vi "2023_day13_Task2.vi"() -> ()   [LabVIEW 2021]
panel:
  out "Task 2":i32
  in  "Switch":bool caption="Ex. Data  vs.  User Data"
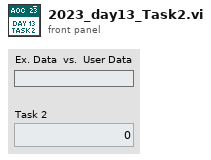
[diagram p1: front panel]
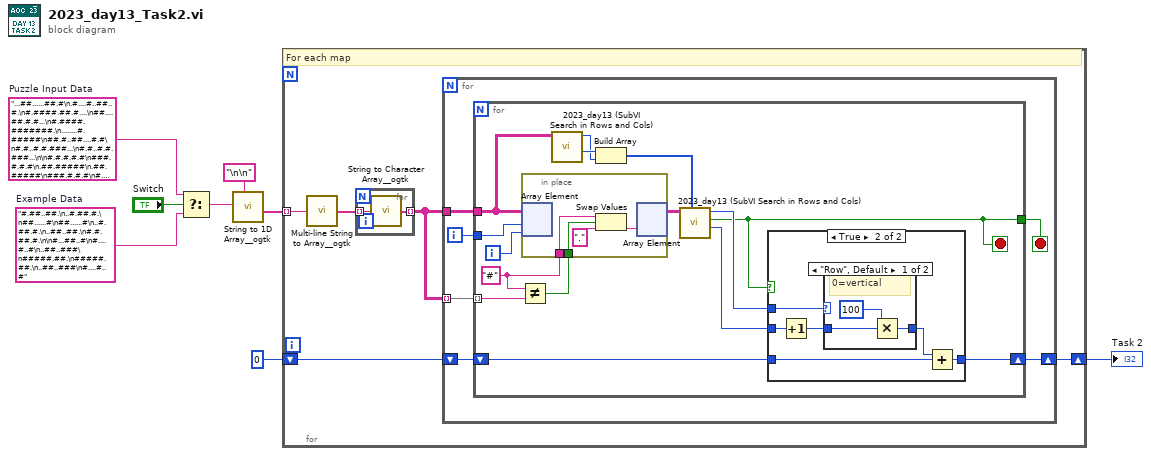
[diagram p0: block diagram]
diagram:
  w6 = "...##......##.#\n.#....#..##..#.\n#.####.##.#....\n##....##.#.#...\n#.####.#######.\n........#.#####\n##.#..##....#.#\n#.#..#.#.###...\n#.#..#.#.###...\n\n#.#.#.#.#\n###.#.#.#\n.##.#####\n.##.#####\n###.#.#.#\n#.#.#.#.#\n.#.##.#.#\n#.#..#..#\n..###.#..\n#..#.#.#.\n##.#...#.\n\n##.....#...\n##.....#...\n#..###....#\n##.#..#.##.\n#..#####..#\n#.#....#.#.\n.##.##....#\n.###..###.#\n...#.......\n....#.#.###\n#......#.##\n...#.##....\n...#.##....\n#......#.##\n....#.#.###\n...#.......\n.###..#####\n\n..####....#\n..####....#\n..#....#.##\n.....#.#..#\n#.#...##...\n###.###.##.\n..#..#...##\n..#..#...##\n###.###.##.\n#.#...##...\n.....#.#..#\n..#.#..#.##\n..####....#\n\n#.#####..\n#..#.#.#.\n.##.#..#.\n.##...##.\n.....#.##\n........#\n........#\n\n..#.###.##..#\n.##.###.##..#\n.#...#.#.#.##\n.#...#.#.#.##\n.##.###.##..#\n..#.###.##..#\n...#.#####.#.\n##.#...######\n..#..#..##.#.\n#..####.###.#\n.##..#....###\n\n####.##....\n....##.##.#\n...##...##.\n##..#..#..#\n##..#....#.\n##..#....#.\n##..#..#..#\n...##...##.\n....##.##.#\n####.##....\n##..#####..\n#..#....#..\n...#.....##\n....#####..\n########...\n#######.#.#\n####.#.#...\n\n..##.......\n#..##.#..#.\n.##....##..\n.#####....#\n#######..##\n.#...##..##\n..####.##.#\n#####..##..\n##.....##..\n##.....##..\n.####..##..\n\n#.#..###.#.##.#\n##.##.###.#..#.\n##...#..#......\n.##...##...##..\n##...###.#.##.#\n.##...#..######\n.#.###.....##..\n...###....#..#.\n#..##..##.#..#.\n#..##..##.#..#.\n...###....#..#.\n.#.###.....##..\n.##......######\n\n#.####.\n#..##..\n##.##.#\n...##..\n#.#..#.\n#####.#\n..#..#.\n..#..#.\n#####.#\n#.#..#.\n...##..\n##.##.#\n#..##..\n#.####.\n..####.\n\n..##.####.#..#.##\n..##..###.#..#.##\n....###..#.##.#..\n......##.######.#\n#.#.#.#..#....#..\n##..###...####...\n#..##..#.#....#.#\n\n##.##..##\n##...##.#\n####.#...\n####.#...\n##...##.#\n##.##..##\n.####.##.\n.##.#...#\n....#....\n#.#..#...\n#.#..#..#\n\n##.##.#..#.\n.#.###....#\n#.#####..##\n#.#####..##\n#....#.....\n##..#######\n.####......\n##.#.######\n##.#.######\n.####......\n##..#######\n\n####.##..\n#..##..##\n.....##..\n#..######\n####.##.#\n####....#\n.##..##..\n####....#\n#..##..##\n.##.#..#.\n#..#.##.#\n.##......\n....####.\n.##..##..\n.....##..\n\n....##..#.#....\n....##..#.#....\n#####.#.#..###.\n.##.#.###.####.\n#.....#..#..###\n.##....#.#....#\n.##.##.#..##..#\n\n.##....##.##..#\n.##.#.#..#...#.\n#..#.#######...\n#..####.##.#..#\n#.##.##.##..#.#\n#..#..#.##..###\n#..#..#.##..###\n\n######...##\n.#####...##\n#.#####..##\n#.#.#.#.#..\n###.#..#...\n..#.....##.\n#....##.##.\n#....##.##.\n..#.....##.\n###.#..#...\n#.#.#.#.#..\n\n...##.....#\n.##...##...\n.##...##...\n.##...##...\n.##...##...\n...##.....#\n.#######.#.\n#...#..##..\n.....##.#.#\n.#.#.#.###.\n.#.#.#.###.\n.....##.#.#\n#...#..##..\n.##.####.#.\n...##.....#\n\n.##.##.\n.##...#\n....###\n#..#...\n#..#.##\n.....##\n#..##..\n.#...##\n#..#.##\n.##.##.\n.##..##\n.##..##\n.##.##.\n\n.##.###........\n##.#.####.##.##\n.####...#.##.#.\n#.##......##...\n...###...####..\n.#.......#..#..\n.#.#..#...##...\n\n##..##.##..#.\n.####......#.\n......#.#####\n.####...#.#..\n.#..#.#.##..#\n#.##.##.#.##.\n.#..#..#..##.\n######.#.#...\n#....###...#.\n#....###...#.\n######.#.#...\n.#..#..##.##.\n#.##.##.#.##.\n\n###..####\n##.##.###\n.######..\n...##....\n...##....\n.#....#..\n##....###\n.##..##..\n##....###\n###..##..\n#.#..#.##\n\n..##..##.\n.#.#.##.#\n.###.##.#\n..##..##.\n..#.#.#..\n#.##....#\n..####..#\n###..#.##\n#...##...\n#...##...\n###..#.##\n\n####.##.#######\n#...####...####\n##.######.#####\n##.######.##...\n..#......#...##\n###.####.######\n####...######..\n#..#.##.#..####\n#.##.##.##.##..\n.##.####.##.#..\n#....##....####\n..#.#..#.#...##\n##..####..##...\n\n...#.#.....##..\n####.#.#.......\n#.#....##..##..\n..#..#.....##..\n.##.#...#..##..\n#.#..##........\n...##..########\n#######.#..##..\n##.####..######\n###...###.####.\n#........######\n.#.##..........\n..##..#.###..##\n.#.#.#..#..##..\n.....###.##..##\n#...#.##.......\n##..##..#......\n\n#..###.....##\n...#...#...##\n##.#.##.....#\n..###..###.##\n.###..##...##\n###.#######..\n#.###...##..#\n#..##...##..#\n###.#######..\n.###..##...##\n..###..###.##\n##.#.##.....#\n...#...#...##\n#..###.....##\n.#.##.##.##..\n.#.##.##.##..\n#..###.....##\n\n##...##.#..#.\n##...##......\n###..##..##..\n###.#........\n....#########\n....#########\n###.#........\n###..##..##..\n#....##......\n##...##.#..#.\n##...#..####.\n..#.##.......\n#.##.########\n#.#.##.##..##\n##...#..####.\n\n.#.##....##.##.\n#####.####..#.#\n.#....##..###.#\n.#...#######..#\n..##.##.#....#.\n...#.#..##.#..#\n...#.#..##.#..#\n..##.##.#....#.\n.#.#.#######..#\n.#....##..###.#\n#####.####..#.#\n.#.##....##.##.\n...#.#.##.##...\n..#.#.#.#.#.###\n##...#.#.....##\n##...#.#.....##\n..#.#.#.#.#.###\n\n..#....#....##...\n##..##..#########\n.#......#.##..##.\n###.##.###..##..#\n##############.##\n.########.#.##.#.\n#..####..#.####.#\n...#..#..........\n#.######.##.##.##\n.##....##...##...\n#..####..#..##..#\n\n#.##.#####.##..#.\n#....#.###...##..\n#....#.##..###..#\n#....#.##..###...\n#....#.###...##..\n#.##.#####.##..#.\n#######..#.####..\n.........#..#....\n########.#...#.##\n#....#.###..#.##.\n##..###..#.#..###\n#....#...###.....\n.####..#.#.#.....\n######..##....###\n######.###...#.#.\n\n.#..#.########.#.\n.####..######..#.\n#....##......##..\n.####.#..##..#.##\n##..#####..#####.\n######..#..#..###\n#########..######\n.####...#..#...##\n######...##...###\n#....#..#..#..#..\n......###..###...\n.#..#.#.####.#.#.\n#.##.##.####.##.#\n.####.#......#.##\n##..##.##..##.##.\n\n.##.#.#..\n#.###....\n###......\n...#.####\n##...##..\n##..#..##\n###.#....\n###.#....\n##..#..##\n##...##..\n...#.####\n###......\n#.###.#..\n.##.#.#..\n.######..\n\n####....##.##.#\n..##.##..##.#.#\n..##.##..##.#.#\n####..#.##.##.#\n..##.#........#\n#.....##....###\n#.#..##...#....\n.###..#..##.##.\n#..#.#.#..##.#.\n##.####.#####..\n..##..#.##...##\n#.##...##.#.#.#\n#..#.##..###..#\n#.##.######...#\n#.##.######...#\n\n##.##.##.\n..####...\n..####..#\n########.\n...##...#\n..####..#\n..####..#\n.#....#..\n..####...\n##.##.###\n###..####\n..####..#\n........#\n##....###\n##....###\n..#..#..#\n..####...\n\n..########.\n..########.\n#.#..###..#\n.#...#.....\n..#...#....\n.#.##..#..#\n.#.....#..#\n.....###...\n#..####.##.\n#..####.##.\n.....###...\n.#.....#.##\n.#.##..#..#\n..#...#....\n.#...#.....\n#.#..###..#\n..########.\n\n....##....#\n..###.#..#.\n.###.######\n.###.######\n..###.#..#.\n....##....#\n##..##.##.#\n.###..#..#.\n##...#.##.#\n.##.#######\n..#.##.....\n.###.......\n#######..##\n##.#.##..##\n#..##.####.\n\n..###..#......#\n##..#.##.#..#.#\n...#.##..#..#..\n..###.####..###\n#####.#..####..\n...#..###.##.##\n..#.#.###..#.##\n##..#..########\n..##.#.########\n.....###..##..#\n..#.##.#......#\n####.#.##.##.##\n########.#..#.#\n..####.##.##.##\n..#.##..#....#.\n\n#.####.#.####.#\n..#..#...##.##.\n.##..##.#......\n.##..##.#......\n..#..#..###.##.\n#.####.#.####.#\n########....##.\n.#.##.#..##..##\n.#.##.#.#.##..#\n#..##..#.##...#\n............#.#\n##....###.....#\n#.#..#.#.###.##\n\n..######......#\n.########.##.##\n..#.##.#......#\n..#.##.#......#\n#.#....#.#..#.#\n##.####.######.\n###...####..###\n\n...#.#.##..#...##\n..#.#.#.########.\n....#....##.#....\n##.......#.....##\n##...##...#.#..##\n.#.#####.#....#..\n.....#####.##.#..\n##.#....#..###...\n.#.#.##...####.##\n.....######..##..\n#.##..#....#.##..\n##.....#...###...\n#.##..#..#.##..##\n#.##..#..#.##..##\n##.....#...###...\n\n#.###..##\n.#.#....#\n##.#..#..\n.##.#..##\n####.....\n.###.....\n.#...#.##\n..#...#..\n..#.#####\n.#.#.....\n.#.#.....\n..#.#####\n..#...#..\n.#...#.##\n.###.....\n\n..##...#.##.#...#\n#.#.##...##...##.\n##.....#....#....\n..#.##........##.\n###.##.#.##.#.##.\n##..##..#..#..##.\n########....#####\n.#.....##..##....\n###.##.##..##.##.\n\n##..#.##....#\n.##..###....#\n#.#.#....##..\n#.##.#..####.\n#.#.#.##....#\n#..####......\n#..####......\n#.#.#.##....#\n#.##.#..####.\n#.#.##...##..\n.##..###....#\n\n...###....#\n...###....#\n..##..#.#..\n..#.....#..\n.........#.\n###..#.##.#\n##.#..#.###\n.#.........\n###.##..#..\n..#.##.####\n##...###.##\n##..#...#..\n##.#.##.##.\n....#..##..\n...#.#####.\n\n.####..#.##..##..\n.###....###..##..\n#.#.#..#.#.#....#\n#####..#####.##.#\n##.##..##.##.##.#\n###......####..##\n##.#.##.#.##.##.#\n\n.#....##.#....#\n.#.##.#.#####..\n###..#.###.###.\n#...#.#.#..###.\n.##.##..#....#.\n###.#.#.#.##..#\n###..#..#..#.#.\n###..#..#..#.#.\n###.#.#.#.##..#\n.##.##..#....#.\n#...#.#.#..###.\n###..#.###.###.\n.#.##.#.#####..\n.#....##.#...##\n.#....##.#...##\n\n###...#..#.#.#.\n.....#.####.#.#\n####..#.#..#.##\n#.#..##.###.###\n##.#####.###.##\n##.#####.###.##\n#.#..##.###.###\n###...#.#..#.##\n.....#.####.#.#\n###...#..#.#.#.\n...#.###.#...##\n.##.#......####\n.##.#......####\n...#.###.#...##\n###...#..#.#.#.\n\n..######..#\n###.##.####\n##.####.##.\n.##....##.#\n##.####.###\n...#..#...#\n###....###.\n..#.##.#..#\n..##..##...\n..##..##...\n##..##..##.\n...#..#....\n###.##.####\n##.####.##.\n....##....#\n\n##.#....#.#\n..#......#.\n##...##...#\n##........#\n##.######.#\n..##.##.###\n...######..\n....#..#...\n..#.####.#.\n..#.#..#.#.\n###.####.##\n...#.##.#..\n##..#..#..#\n..#..##..#.\n##.######.#\n\n###.##..#\n.#####..#\n....#....\n###...##.\n##.##.##.\n####.....\n..###....\n\n##.##.##.##\n##.########\n...#......#\n####..##..#\n##..#....#.\n###.######.\n##.##....##\n##.#..##..#\n##.#.####.#\n##..#....#.\n######..###\n##.........\n###..####..\n..#.#.##.#.\n###..#..#..\n...###.####\n#####.##.##\n\n.#..######..#..#.\n#..###..###..##..\n#...######...##..\n..###....#.#....#\n#....####....##..\n.##..####..##..##\n.#.##....##.#..#.\n###.#.##.#.######\n##..##..##..####.\n#.#..#..#..#.##.#\n...#..##..#......\n\n##.#..#\n###...#\n.###.##\n.###.##\n###...#\n##.#..#\n..#..##\n##..#..\n.#.....\n.#.....\n##..#..\n#.#..##\n##.#..#\n\n####.#.\n..#...#\n##...#.\n..#..##\n###.##.\n....#..\n##.####\n##....#\n..#####\n..#####\n##....#\n##.####\n....#..\n###.##.\n..#..##\n##...#.\n..#.#.#\n\n..##.###.##.###\n#..#.##.####.##\n##.##..######..\n###..##.####.##\n.####..........\n..##..########.\n.##..##......##\n.##..##......##\n..##..########.\n.####..........\n###..##.####.##\n##.##..######..\n#..#.##.####.##\n..######.##.###\n#....#.#.##.#.#\n\n#####..\n##.#.##\n..#####\n.##..##\n..#..##\n...#.##\n##.##..\n.####..\n##.....\n.#..#..\n.#..#..\n##.....\n..###..\n##.##..\n...#.##\n\n..####.##.#\n.#.##.#..#.\n.#....#....\n.######...#\n##.##.##...\n.######...#\n.#....#.##.\n###..###..#\n##....#####\n..#..#...#.\n..#..#...#.\n\n###..#.\n...###.\n.##.###\n.#####.\n##..###\n.###.##\n.#..#..\n..###..\n..###..\n.#..#..\n####.##\n##..###\n.#####.\n.##.###\n...###.\n###..#.\n###..#.\n\n..#######\n...######\n...##....\n##.#..###\n..#.#.###\n.##....##\n######...\n#..######\n.#.####..\n.#..##...\n..###....\n.#####.##\n##.###...\n\n...##....##\n...##....##\n#.####.#...\n.#.##.#.##.\n.#....#.###\n.######..#.\n.........##\n..####....#\n.#....#...#\n...##...#.#\n##.##.####.\n#..##.##...\n#.#..#.##..\n\n######...#....#\n..##...........\n..##..#.##.##.#\n##..####.#.##.#\n#.##.##.#.####.\n.####..##.####.\n########.######\n#.##.##.###..##\n.#..#..#.#.##.#\n.####.#.#......\n#.##.#...####.#\n\n#...#.###\n.###..##.\n..##.#.##\n.##.#.#..\n..#.##.#.\n.#..#..#.\n.#.#.#.##\n.#.###.##\n.#..#..#.\n.#..#..#.\n.#.###.##\n.#.#.#.##\n.#..#..#.\n\n....#.##..###\n#######.#.#..\n##.#..##.....\n####.#.#.#.##\n#####......##\n...###.###.#.\n......####.##\n\n.#..###..###..#..\n.#.#..#..#..#.#..\n.#..##.##.##..#..\n.......##........\n##.##.#..#.##.###\n###..######..####\n##.##.#.##.##.###\n#.#..######..#.##\n..#...####...#...\n\n#....#....#\n.####....#.\n#....##.#..\n#....####..\n.####....#.\n#....#....#\n.####....##\n\n########.\n##.##.###\n...##...#\n..####..#\n#.#..#.#.\n##....###\n##....###\n###..###.\n###..###.\n...##...#\n...##...#\n..####...\n........#\n\n#.###..##\n##...##..\n#.#......\n#....##..\n#....##..\n..#.####.\n..#......\n\n..#..###...#.\n..#..###...#.\n...##...##.##\n##....##...#.\n##.##.##.#..#\n...######...#\n..#..#...#.##\n##...##..#...\n#..#.##..#..#\n....#.#.#.##.\n###..#.#.##.#\n\n#..#...\n...##.#\n.#.....\n..#.#.#\n..#.#.#\n.#.....\n...####\n#..#...\n#.#.#.#\n#.#.#.#\n#..#...\n...####\n.#.....\n\n..##.####.##...##\n..##.####.##...##\n..#..#..#..#..##.\n.##.##..##.##.#..\n#...##..##...#.#.\n#.##......##.#.#.\n.##..#..#..##.#..\n#...##..#....####\n######..#######.#\n.###.####.###..#.\n.##..####..##.#..\n\n##.#.######..#.##\n.##..#..#.###.#..\n#####..#####...##\n#####..#####...##\n.##..#..#.###.#..\n##.#.######..#.##\n.##.###....###.##\n.##..####..#....#\n.##.####.#.#.####\n..#..#.#...####..\n.###...######.###\n\n...#.#.###.\n...#.#.###.\n###...##.##\n......##..#\n#.#..#..#..\n.#.#..#...#\n##.##..##..\n#..#.#..##.\n#..###..#..\n#.####..#..\n#..#.#..##.\n\n#.#....#...\n.#.###.###.\n..##.##...#\n.#..###..##\n..#...#..##\n..#...#..##\n.#..###..##\n..##.##...#\n.#.##..###.\n#.#....#...\n...#####...\n...#####...\n#.#....#...\n.#.##..###.\n..##.##...#\n\n#.#####..#.#.#.#.\n##..#..#.##.##..#\n..##......#...#..\n####...###.#.#.#.\n...#.#.#....#####\n....#....##.##.#.\n....#....##.##.#.\n#..#.#.#....#####\n####...###.#.#.#.\n..##......#...#..\n##..#..#.##.##..#\n#.#####..#.#.#.#.\n#.#####..#.#.#.#.\n\n#.#..##..##.#\n##..#...###..\n#.##.#....#..\n#.##.#....#..\n##..#...###..\n#.#..##..#..#\n##.##.#..#..#\n...#######.#.\n.###.##....##\n.#.#....#...#\n.##.##..##...\n###.#.#.#.###\n###.#...###..\n.#.###.....#.\n#.#.####..##.\n#.#.####..##.\n.#.###.....#.\n\n.##..#.####..\n.#.#.#.######\n#.###..###...\n#..##.#.#####\n###..#.#.#.#.\n#.##.#.##.###\n...#.###.####\n##.#.##....##\n##.#.##.#..##\n.#.#..####.##\n##.###..#..#.\n##.###..#..#.\n.#.#..####.##\n##.#.##.#..##\n##.#.##....##\n\n#...##..#\n#####....\n#####....\n#...##..#\n.#....###\n.#.#..###\n#...##..#\n\n#......##\n#......#.\n.##..##..\n.##..##..\n#......##\n###..####\n#......##\n#.#..#.##\n##.##.###\n..#..#..#\n........#\n..####...\n.#.##.#..\n........#\n........#\n.#.##.#..\n.######..\n\n#........#..#..#.\n##..##..##..##..#\n#..####..####..##\n#.#....#.#..#.#..\n.#......#.##.#...\n.##....##.##.##..\n##.#..#.######.#.\n###.##.########.#\n..#....#..##..#..\n\n..........###..##\n####..#######.#..\n##.#..#.###....##\n#........#.###...\n####..####.#...##\n.##....##.##.#...\n##.####.##..###..\n###.##.###...##..\n##.####.##.##.###\n.#..##..#.###..##\n##..##..###.##...\n.########.#.##.##\n.#.####.#...###..\n.###..###.#######\n#.#.##.#.##...#.#\n..#.##.#..##.#.##\n#........###.##..\n\n..#.###\n.#.....\n..#.##.\n..#.##.\n.#.....\n..#.###\n#.####.\n.##...#\n.#.###.\n.#.###.\n.#....#\n\n#..###.\n####..#\n####..#\n#..###.\n.##.##.\n###.###\n...####\n...####\n###.###\n.#..##.\n#..###.\n\n#....#...#...\n#....#.####.#\n#....#.####.#\n#....#...#...\n......######.\n.####.#..##.#\n#######..#.##\n.##.#..##.#.#\n#....######.#\n\n..#....#.##..##\n.#....####.##..\n.#.##...#######\n#.##..###......\n#.#.....#######\n##.#.....######\n###...##...##..\n..##..##.#....#\n###.##...#....#\n..###.##.......\n#.##...##......\n.##...###.#..#.\n.##...###.#..#.\n#.##...##......\n..###.##.......\n###.##...#....#\n..##..##.#....#\n\n....#...#.#.#..\n##...#.#.#.....\n.####.##.......\n.......#.#.##.#\n#..#..#.#..#.#.\n#..##.#.#..#.#.\n.......#.#.##.#\n.####.##.......\n##...#.#.#.....\n....#...#.#.#..\n....#...#.#.#..\n\n#..####..#..#\n#..#..#..####\n#..#.....#..#\n##..##..#####\n#..####..#..#\n##..##..##..#\n.###..###....\n\n..#....##\n...##..#.\n...######\n##.#.#..#\n######.#.\n......#.#\n#####.##.\n...##....\n##.##.##.\n...##....\n##..#####\n##..#####\n...##..#.\n##.##.##.\n...##....\n#####.##.\n......#.#\n\n####.###.\n####..#..\n####..#..\n####.###.\n#..#.####\n......##.\n#..#.##..\n....#.##.\n#..#..###\n##.##..##\n.##......\n\n###.#.#.#\n###.#.#.#\n...#.#.##\n#.##..#..\n#.###.##.\n#.####.#.\n##.######\n#.##..#..\n#.##..#..\n##.######\n#.####.#.\n#.######.\n#.##..#..\n...#.#.##\n###.#.#.#\n\n...#.#.##.#\n...#.#.##.#\n#.#.#.#...#\n#.###...##.\n#..##.##.##\n##..####.#.\n##..####.#.\n#..##.##.##\n#.####..##.\n\n#.#.#.##.###.\n..##.#..##...\n..##.#..##...\n..#.#.##.###.\n.#.#.##....#.\n..#.#.###.#.#\n..#.#.###.#.#\n\n...#......#..\n##...#..#...#\n###..#..#..##\n...#.####.#..\n..##.#..#.##.\n....######...\n....##...#...\n\n....#.##.########\n.####.##.##......\n..##..###.#.#.#.#\n########....#.##.\n..##......#.#.##.\n.#..#...#..###.##\n.#..#...#..###.##\n\n##...#..###\n..##....###\n....#..#...\n#####..#...\n##.#..####.\n##.#..####.\n#####..#..#\n\n#.###..##.###..\n#....#..##.####\n#.#####.##.#...\n..#####.....#..\n###.####..#####\n##.#.....#.#...\n#.#....##..####\n##..#...#..##..\n.#...#.#..##.##\n##..#.##.##.#..\n#.#.#####.#....\n##..##.#..#....\n.#..##.....##..\n#..#...#...#...\n#.##...#...#...\n..##.#....#.###\n..##.#...##.###\n\n##..###..#.####\n.###.#.##..####\n###...#..#.....\n.........##.##.\n..#....##.#.##.\n###...#...#....\n..#..#....##..#\n#.....#.##.....\n#...#...#......\n.#..##..###....\n.#.###..###....\n\n.##.#..#.....\n########.....\n###..#...####\n####.#.##.##.\n......#.#.##.\n#..#.##.#.##.\n####.##.#####\n.....#..#####\n.##..##.#.##.\n.##...##.####\n.....##.#####\n.##....###..#\n.##.#.#...##.\n.##.#.#......\n#..#..##..##.\n....##.......\n####.#..#....\n\n.###.##.#\n.###.##.#\n##.#.....\n####.##.#\n##...####\n....###..\n.#....#..\n#..#.####\n#..#.####\n.#...##..\n....###..\n##...####\n####.##.#\n##.#.....\n.###.##.#\n\n...#.######\n...#.######\n#.#.#.#....\n###...##...\n##.########\n...#.#.....\n...##.#.##.\n.#...###..#\n..####.####\n.#.#.#.....\n#......####\n\n######...#...\n#.##.##.#####\n######...#...\n.#..#..#####.\n......###..#.\n..##....#.#..\n..##..#.##.##\n..##..#.##.##\n..##....#.#..\n......###..#.\n.#..#..#####.\n######...#...\n#.##.#..#####\n######...#...\n#.##.#.#..###"  # Puzzle Input Data
  w7 = "#.##..##.\n..#.##.#.\n##......#\n##......#\n..#.##.#.\n..##..##.\n#.#.##.#.\n\n#...##..#\n#....#..#\n..##..###\n#####.##.\n#####.##.\n..##..###\n#....#..#"  # Example Data
  n1 = Select(t=w6, s="Switch", f=w7) -> (s? t:f=w5:string)
  n2 = call <userlib>:"String to 1D Array__ogtk.vi"("delimiter (Tab)"="\n\n", "string"=w5) -> ("Array of Strings"=w3:string[])  [unwired: 9 in]
  n3 = for {
    tunnel: w3 -> [w13] mode=indexing
    shift-right: [w10] -> w1
    shift-left: 0 -> [w11]
    # "For each map"
    n4 = call <userlib>:"Multi-line String to Array__ogtk.vi"("string"=w13) -> ("lines"=w12:string[])
    n5 = for {
      tunnel: w12 -> [w51] mode=indexing
      tunnel: [w50] -> w9 mode=indexing
      n6 = call <userlib>:"String to Character Array__ogtk.vi"("Input String"=w51) -> ("Character Array"=w50:string[])
    }
    n7 = for {
      shift-right: [w18] -> w10
      shift-left: w11 -> [w19]
      tunnel: w9 -> [w17] mode=indexing
      tunnel: w9 -> [w15]
      i -> [w16]
      stop <- w14 stop-if-true
      n8 = for {
        shift-right: [w33] -> w18
        shift-left: w19 -> [w34]
        tunnel: w17 -> [w30] mode=indexing
        tunnel: w16 -> [w32]
        tunnel: w15 -> [w24]
        tunnel: [w20] -> w14
        i -> [w31]
        stop <- w20 stop-if-true
        w28 = "#" ("String")
        n9 = Not Equal?(x=w28, y=w30) -> (x != y?=w29:bool)
        n10 = in-place {
          in-place-border: w29 -> [w48]
          in-place-border: w28 -> [w47]
          n11 = in-place-array #1(w24, w32, w31) -> ()  [unwired: 1 out]
          n12 = Swap Values(12:w47, 13:w48, 14:"." ("String")) -> (3:w49:string)  [unwired: 1 out]
          n13 = in-place-array #1(w49) -> (w27:string[][])  [unwired: 2 out]
        }
        n14 = call "2023_day13 (SubVI Search in Rows and Cols).vi"("Character Array"=w24) -> ("Match Index"=w23:i32, "Row or Col"=w22:enum32{"Row", "Col"})  [unwired: 8 in, 1 out]
        n15 = Build Array(w23, w22) -> (w21:u32[])
        n16 = call "2023_day13 (SubVI Search in Rows and Cols).vi"("Ignore Case"=w21, "Character Array"=w27) -> ("Match Index"=w26:i32, "Match Found?"=w20:bool, "Row or Col"=w25:enum32{"Row", "Col"})  [unwired: 7 in]
        n17 = case shown="True" w20 {
          tunnel: w34 -> [w35 w40]
          tunnel: [w35 w39] -> w33
          tunnel: w26 -> [_ w37]
          tunnel: w25 -> [_ w36]
          frame False {
          }
          frame True {
            n18 = Increment(x=w37) -> (x+1=w38:i32)
            n19 = case shown="\"Row\", Default" w36 {
              tunnel: w38 -> [w44 w45]
              tunnel: [w42 w45] -> w41
              frame "Row", Default {
                # "0=vertical"
                n20 = Multiply(x=100 ("y"), y=w44) -> (x*y=w42:i32)
              }
              frame "Col" {
                # "1=horizontal"
              }
            }
            n21 = Add(x=w41, y=w40) -> (x+y=w39:i32)
          }
        }
      }
    }
  }
  "Task 2" <- w1
